vi "get channels.vi"(11 "CVT configuration in":refnum<class "CVT configuration.lvclass">) -> (2 "channels":refnum<class "TBM channel.lvclass">[](array[class]), 3 "CVT configuration out":refnum<class "CVT configuration.lvclass">)   [LabVIEW 2013, in "CVT configuration.lvclass"]
uses:
  CVT configuration.lvclass
  <vilib>/NI/Tag Bus Module Framework/channel/TBM channel.lvclass
  CVT configuration.lvclass/CVT configuration.ctl
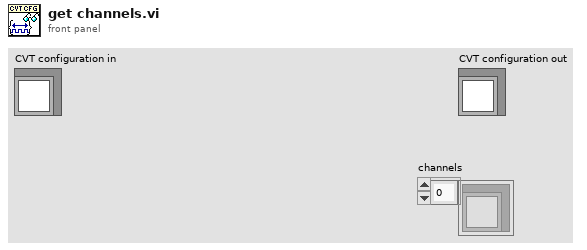
[diagram p1: front panel]
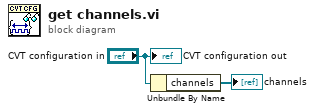
[diagram p0: block diagram]
diagram:
  n1 = Unbundle By Name("CVT configuration in") -> ("channels"=→"channels":refnum<class "TBM channel.lvclass">[])
  "CVT configuration out" <- "CVT configuration in"
